vi "Configure Devices to Load.vi"(9 "Microgrid ID":u8, 10 "Device IDs":T1[](array[typedef]), 11 "Devices to Load in":refnum<class "Devices to Load.lvclass">) -> (3 "Devices to Load out":refnum<class "Devices to Load.lvclass">)   [LabVIEW 2018, in "Devices to Load Config Actor.lvlib" / "Devices to Load.lvclass"]
uses:
  Devices to Load.lvclass
  <vilib>/ORNL/CSEISMIC DDS/CSEISMIC DDS Base/Data Types/Controls/DeviceID.ctl
  Devices to Load.lvclass/Devices to Load.ctl
  <vilib>/ORNL/CSEISMIC DDS/CSEISMIC DDS Base/CSEISMIC DDS.lvclass
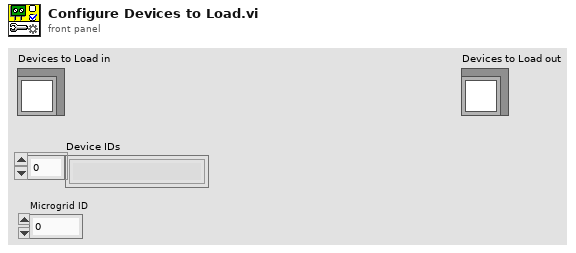
[diagram p1: front panel]
types:
  T1 = typedef "CSEISMIC DDS.lvlib/CSEISMIC DDS.lvclass/DeviceID.ctl" = string
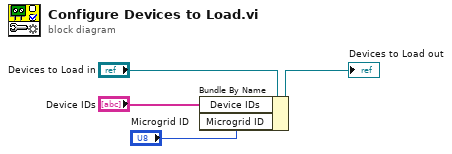
[diagram p0: block diagram]
diagram:
  n1 = Bundle By Name(cluster="Devices to Load in", "Device IDs"="Device IDs", "Microgrid ID"="Microgrid ID") -> (→"Devices to Load out":refnum<class "Devices to Load.lvclass">)
